vi "PH_PILS.Enabling Checking.vi"(0 "i ref in":refnum<vi>, 2 "System to enable":u16(ring) items=["PreAmp", "MainAmp", "ext Exp"], 5 "error in":errorcluster) -> (14 "i ref out":refnum<vi>, 17 "Enabling allowed":bool, 19 "error out":errorcluster)   [LabVIEW 2014, in "PH_PILS.lvlib"]
doc: "This VI checks whether the enabling person is authorized to do it."
uses:
  PH_PILS.lvlib
  PH_Devices/PH_Beckhoff_PPMA-Rods/PH_Beckhoff_PPMA-Rods.Rods Tags.ctl
  PH_Devices/PH_Beckhoff_PPMA-Rods/PH_Beckhoff_PPMA-Rods.lvlib
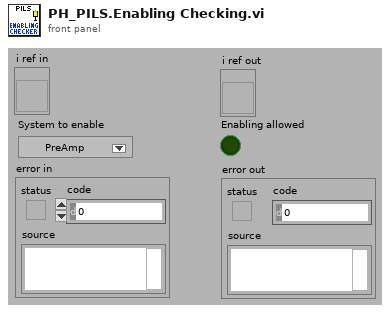
[diagram p1: front panel]
types:
  T1 = typedef "PH_Beckhoff_PPMA-Rods.lvlib/PH_Beckhoff_PPMA-Rods.Rods Tags.ctl" = enum16{"Rod-up", "earth-ok", "door-locked-K1", "door-locked-K2", "watervalve-closed", "Rods-Chain-A-up", "Rods-Chain-B-up", "HV-Warnlamp-orange", "HV-Warnlamp-green", "Status-Rods-PU-1", "Status-Rods-PU-2", "Status-Rods-PU-3", "Status-Rods-PU-4", "Status-Rods-PU-5", "Status-Rods-PU-6", "Status-Rods-PU-7", "Status-Rods-PU-8", "Status-Rods-PU-9", "Status-Rods-PU-10", "Status-Rods-FR", "Status-Rods-PILC"}
  T2 = typedef "PH_PILS.lvlib/PH_PILS.i attribute.ctl" = cluster{"Boolean":cluster{"GUI Ref":refnum<vi>, "Status":i32}[], "GUI Refs Exp. Shutters":cluster{"1":refnum<vi>, "2":refnum<vi>, "3":refnum<vi>, "4":refnum<vi>}, "Tristate2Run GUI Refs":refnum<vi>[], "EO-Likes":cluster{"GUI Ref":refnum<vi>, "Status":i32}[], "Operation Mode":cluster{"Operation Mode":T3, "GUI":cluster{"Ref State":refnum<vi>, "Ref":refnum<vi>}, "Servicemode":cluster{"Tagname":string, "Status":i32}, "Labormode":cluster{"Tagname":string, "Status":i32}, "Searchmode":cluster{"Tagname":string, "Status":i32}, "Shotmode":cluster{"Tagname":string, "Status":i32}}, "Submode":cluster{"Submode":T4, "GUI":cluster{"Ref State":refnum<vi>, "Ref":refnum<vi>}, "Submode":cluster{"Tagname":string, "Status":i32}}, "Experiment":cluster{"Experiment":enum16{"unknown", "intern", "4 (Z6)", "3", "2", "1"}, "GUI":cluster{"Ref State":refnum<vi>, "Ref":refnum<vi>}, "intern":cluster{"Tagname":string, "Status":i32}, "Exp 4":cluster{"Tagname":string, "Status":i32}, "Exp 3":cluster{"Tagname":string, "Status":i32}, "Exp 2":cluster{"Tagname":string, "Status":i32}, "Exp 1":cluster{"Tagname":string, "Status":i32}}, "TristateNormal":cluster{"GUI Ref":refnum<vi>, "Status":i32}[], "Door Tags":cluster{"GUI Ref":refnum<vi>, "Status":i32}[], "GUIlessTags":cluster{"Name":string, "Status":i32}[], "Beamline GUI Refs":refnum<vi>[], "Special Boolean":cluster{"GUI Ref":refnum<vi>, "Status":i32}[], "Laserpower":cluster{"GUI Ref":refnum<vi>, "Status":i32}[], "Shutter":cluster{"GUI Ref":refnum<vi>, "Status":i32}[], "Tristate EO Like":cluster{"GUI Ref":refnum<vi>, "Status":i32}[], "PP":cluster{"GUI Ref":refnum<vi>, "Status":i32, "Head Ref":refnum<vi>, "Slider Ref":refnum<vi>}[], "Switch Knobs":cluster{"GUI Ref":refnum<vi>, "Status":i32}[], "Latch Knob GUI Refs":refnum<vi>[], "FailureCounter":i32, "Enabled Status":cluster{"Laser":i32, "PreAmp":i32, "MainAmp":i32}, "Mercury":refnum<vi>, "Instance Rods":string, "Logfile":path, "Beckhoff-Instance Internal":string, "Beckhoff-Instance External":string, "Enabling Rights":cluster{"Name":string, "Password":string, "PA?":bool, "MA?":bool, "Exp?":bool}[]}
  T3 = typedef "PH_PILS.lvlib/PH_PILS.Operation Mode.ctl" = enum16{"unknown", "Service", "Labor", "Search", "Shot"}
  T4 = typedef "PH_PILS.lvlib/PH_PILS.Submode.ctl" = enum16{"unknown", "HV-Normal", "HV-Test"}
  T5 = cluster{"Name":string, "Password":string, "PA?":bool, "MA?":bool, "Exp?":bool}[]
  T6 = cluster{"Name":string, "Password":string, "PA?":bool, "MA?":bool, "Exp?":bool}
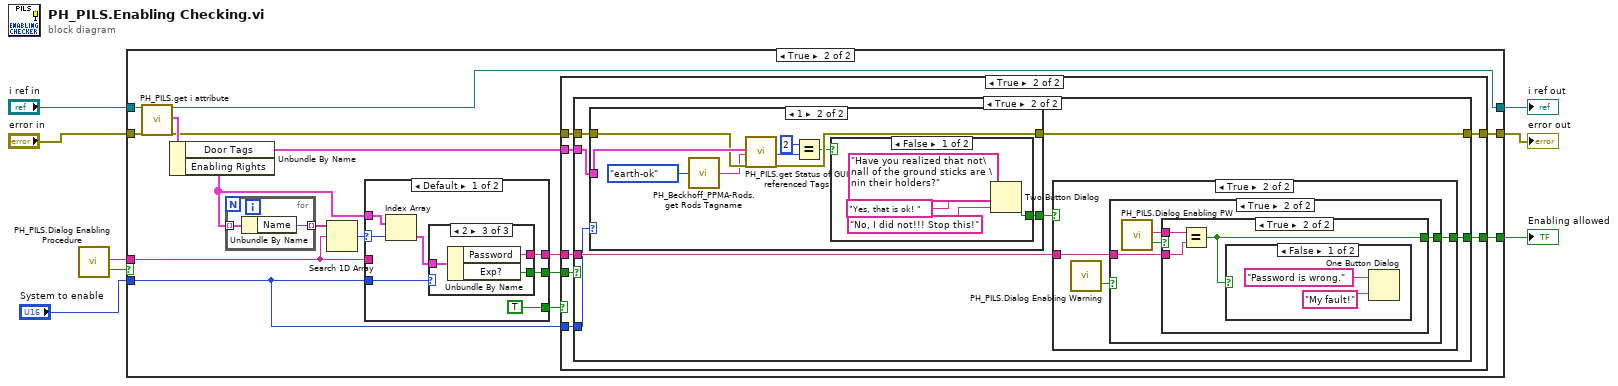
[diagram p0: block diagram]
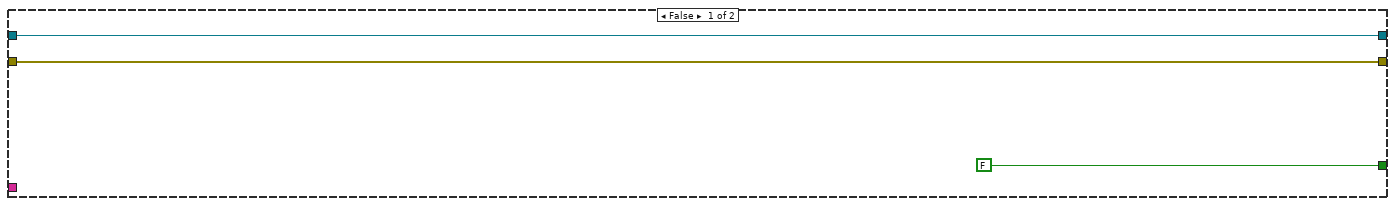
[diagram p2: hidden frame]
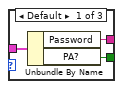
[diagram p3: hidden frame]
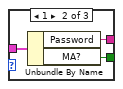
[diagram p4: hidden frame]
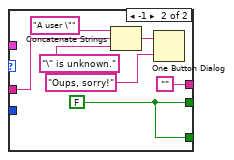
[diagram p5: hidden frame]
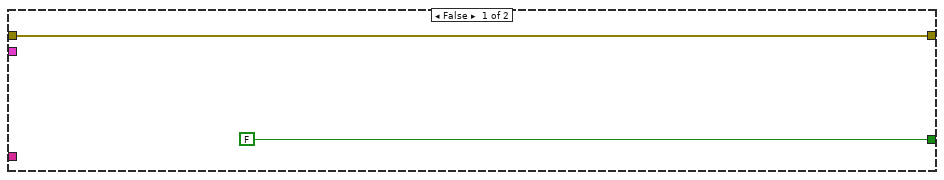
[diagram p6: hidden frame]
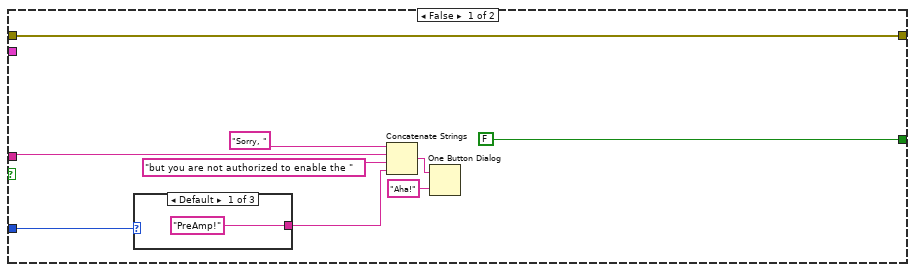
[diagram p7: hidden frame]
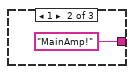
[diagram p8: hidden frame]
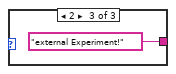
[diagram p9: hidden frame]
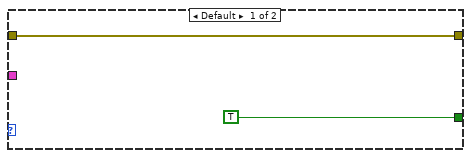
[diagram p10: hidden frame]
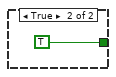
[diagram p11: hidden frame]
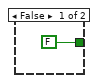
[diagram p12: hidden frame]
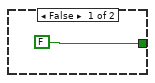
[diagram p13: hidden frame]
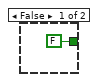
[diagram p14: hidden frame]
diagram:
  n1 = call "PH_PILS.Dialog Enabling Procedure.vi"() -> ("User Name"=w5:string, "o.k."=w3:bool)  [unwired: 18 in]
  n2 = case shown="True" w3 {
    tunnel: [w10 w15] -> w8
    tunnel: "i ref in" -> [w10 w13]
    tunnel: "error in" -> [w9 w12]
    tunnel: w5 -> [_ w23]
    tunnel: [FALSE w27] -> w4
    tunnel: [w9 w16] -> w2
    tunnel: "System to enable" -> [_ w19]
    frame False {
    }
    frame True {
      n3 = call "PH_PILS.get i attribute.vi"("i ref in"=w13, "error in (no error)"=w12) -> ("i ref out"=w15:refnum<vi>, "i attribute"=w26:T2, "error out"=w17:errorcluster)  [unwired: 15 in]
      n4 = Unbundle By Name(w26) -> ("Door Tags"=w18:cluster{"GUI Ref":refnum<vi>, "Status":i32}[], "Enabling Rights"=w14:T5)
      n5 = for {
        tunnel: w14 -> [w52] mode=indexing
        tunnel: [w51] -> w25 mode=indexing
        n6 = Unbundle By Name(w52) -> ("Name"=w51:string)
      }
      n7 = Search 1D Array(1D array=w25, element=w23) -> (index of element=w24:i32)  [unwired: 1 in]
      n8 = case shown="Default" w24 {
        selector: w24 -> [w33 _]
        tunnel: [TRUE w44] -> w22
        tunnel: w23 -> [_ w46]
        tunnel: [w30 ""] -> w21
        tunnel: w14 -> [w34 _]
        tunnel: [w29 w44] -> w20
        tunnel: w19 -> [w28 _]
        frame Default {
          n9 = Index Array(array=w34, index=w33) -> (element=w31:T6)
          n10 = case shown="2" w28 {
            tunnel: w31 -> [w37 w40 w43]
            tunnel: [w36 w39 w42] -> w30
            tunnel: [w35 w38 w41] -> w29
            frame Default {
              n11 = Unbundle By Name(w37) -> ("Password"=w36:string, "PA?"=w35:bool)
            }
            frame 1 {
              n12 = Unbundle By Name(w40) -> ("Password"=w39:string, "MA?"=w38:bool)
            }
            frame 2 {
              n13 = Unbundle By Name(w43) -> ("Password"=w42:string, "Exp?"=w41:bool)
            }
          }
        }
        frame -1 {
          w44 = FALSE
          n14 = Concatenate Strings("A user \"" ("string"), w46, "\" is unknown." ("string")) -> (w48:string)
          n15 = One Button Dialog(message=w48, button name ("OK")="Oups, sorry!") -> ()  [unwired: 1 out]
        }
      }
      n16 = case shown="True" w22 {
        tunnel: w21 -> [_ w60]
        tunnel: [FALSE w61] -> w27
        tunnel: w20 -> [_ w59]
        tunnel: w19 -> [_ w58]
        tunnel: w18 -> [_ w57]
        tunnel: w17 -> [w53 w56]
        tunnel: [w53 w55] -> w16
        frame False {
        }
        frame True {
          n17 = case shown="True" w59 {
            tunnel: [FALSE w80] -> w61
            tunnel: w60 -> [w66 w79]
            tunnel: w58 -> [w65 w77]
            tunnel: w57 -> [_ w78]
            tunnel: w56 -> [w62 w76]
            tunnel: [w62 w75] -> w55
            frame False {
              n18 = case shown="Default" w65 {
                tunnel: ["PreAmp!" ("button name (\"OK\")") "MainAmp!" ("button name (\"OK\")") "external Experiment!" ("button name (\"OK\")")] -> w64
                frame Default {
                }
                frame 1 {
                }
                frame 2 {
                }
              }
              n19 = Concatenate Strings("Sorry, " ("string"), w66, "but you are not authorized to enable the " ("string"), w64) -> (w68:string)
              n20 = One Button Dialog(message=w68, button name ("OK")="Aha!") -> ()  [unwired: 1 out]
            }
            frame True {
              n21 = case shown="1" w77 {
                tunnel: w78 -> [_ w89]
                tunnel: w76 -> [w82 w88]
                tunnel: [w82 w87] -> w75
                tunnel: [TRUE w85] -> w74
                frame Default {
                }
                frame 1 {
                  n22 = call "PH_Beckhoff_PPMA-Rods.get Rods Tagname.vi"("Rods Tag"=PH_Beckhoff_PPMA-Rods.Rods_Tags."earth-ok") -> ("Rods Tagname"=w83:string)
                  n23 = call "PH_PILS.get Status of GUI referenced Tags.vi"("Tags"=w89, "Tagname"=w83, "error in"=w88) -> ("Status"=w90:i32, "error out"=w87:errorcluster)  [unwired: 13 in, 2 out]
                  n24 = Equal?(x=2, y=w90) -> (x = y?=w86:bool)
                  n25 = case shown="False" w86 {
                    tunnel: [w92 TRUE] -> w85
                    frame False {
                      n26 = Two Button Dialog(message="Have you realized that not\nall of the ground sticks are \nin their holders?", 1:"No, I did not!!! Stop this!" ("F button name (\"Cancel\")"), 2:"Yes, that is ok! " ("T button name (\"OK\")")) -> (T button?=w92:bool)
                    }
                    frame True {
                    }
                  }
                }
              }
              n27 = case shown="True" w74 {
                tunnel: [FALSE w100] -> w80
                tunnel: w79 -> [_ w99]
                frame False {
                }
                frame True {
                  n28 = call "PH_PILS.Dialog Enabling Warning.vi"() -> ("o.k."=w98:bool)  [unwired: 19 in]
                  n29 = case shown="True" w98 {
                    tunnel: [FALSE w105] -> w100
                    tunnel: w99 -> [_ w104]
                    frame False {
                    }
                    frame True {
                      n30 = call "PH_PILS.Dialog Enabling PW.vi"() -> ("User Name"=w103:string, "o.k."=w102:bool)  [unwired: 18 in]
                      n31 = case shown="True" w102 {
                        tunnel: [FALSE w109] -> w105
                        tunnel: w104 -> [_ w108]
                        tunnel: w103 -> [_ w107]
                        frame False {
                        }
                        frame True {
                          n32 = Equal?(x=w107, y=w108) -> (x = y?=w109:bool)
                          n33 = case shown="False" w109 {
                            frame False {
                              n34 = One Button Dialog(message="Password is wrong.", button name ("OK")="My fault!") -> ()  [unwired: 1 out]
                            }
                            frame True {
                            }
                          }
                        }
                      }
                    }
                  }
                }
              }
            }
          }
        }
      }
    }
  }
  "i ref out" <- w8
  "error out" <- w2
  "Enabling allowed" <- w4
